vi "set_result_types.vi"(8 "error in (no error)":errorcluster, 10 "result_types":refnum<class "Type.lvclass">[](array[class]), 11 "FunctionType in":refnum<class "FunctionType.lvclass">) -> (0 "error out":errorcluster, 3 "FunctionType out":refnum<class "FunctionType.lvclass">)   [LabVIEW 2020, in "mlir.lvlib" / "FunctionType.lvclass"]
uses:
  FunctionType.lvclass
  FunctionType.lvclass/FunctionType.ctl
  Type/Type.lvclass
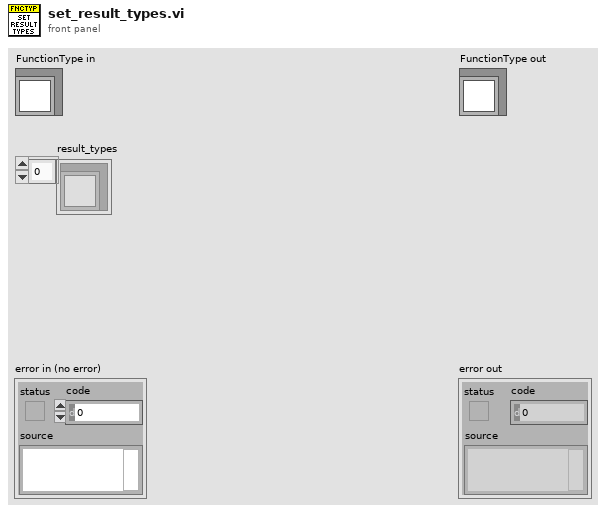
[diagram p1: front panel]
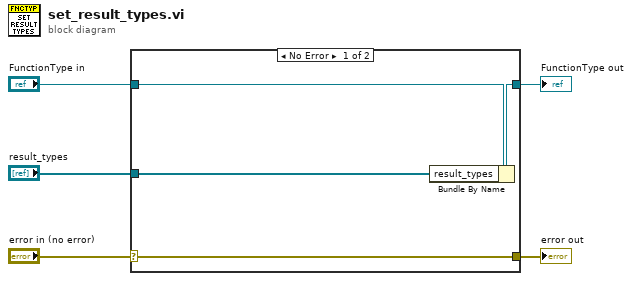
[diagram p0: block diagram]
diagram:
  n1 = case shown="No Error" "error in (no error)" {
    selector: "error in (no error)" -> [w9 w10]
    tunnel: [w9 w10] -> w4
    tunnel: [w7 w11] -> w2
    tunnel: "FunctionType in" -> [w8 w11]
    tunnel: "result_types" -> [w6 _]
    frame No Error {
      n2 = Bundle By Name(cluster=w8, "result_types"=w6) -> (w7:refnum<class "FunctionType.lvclass">)
    }
    frame Error {
    }
  }
  "error out" <- w4
  "FunctionType out" <- w2
